vi "Read Source.vi"(8 "Error In":errorcluster, 11 "Node In":refnum<class "Tag.lvclass">) -> (0 "Error Out":errorcluster, 2 "Source":string, 3 "Node Out":refnum<class "Tag.lvclass">)   [LabVIEW 2018, in "Toolkit.lvlib" / "Nodes.lvlib" / "Tag.lvclass"]
uses:
  Tag.lvclass
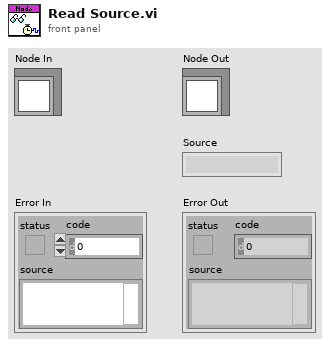
[diagram p1: front panel]
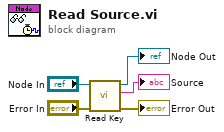
[diagram p0: block diagram]
diagram:
  n1 = call "Read Key.vi"("Error In"="Error In", "Tag In"="Node In") -> ("Error Out"=→"Error Out":errorcluster, "Key"=→"Source":string, "Tag Out"=→"Node Out":refnum<class "Tag.lvclass">)  [unwired: 7 in]
